vi "Parse StdErr for StdOut.vi"(11 "StdErr Event":string) -> (0 "error out":errorcluster, 2 "StdOut":string, 3 "StdErr":string)   [LabVIEW 2020, in "Kasli Wrapper 2.0.lvlib" / "Kasli Wrapper 2.0.lvclass"]
uses:
  Kasli Wrapper 2.0.lvclass
  <vilib>/regexp/Match Regular Expression.xnode
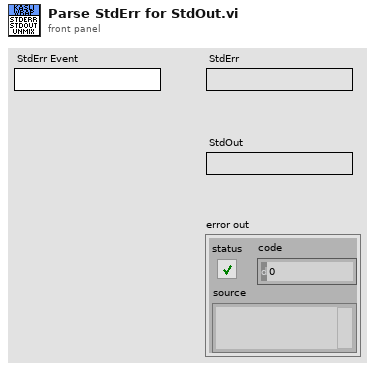
[diagram p1: front panel]
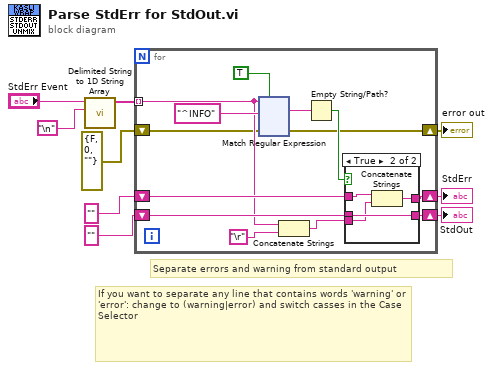
[diagram p0: block diagram]
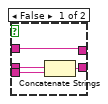
[diagram p2: hidden frame]
diagram:
  # "If you want to separate any line that contains words 'warning' or 'error': change to (warning|error) and switch casses in the Case Selector"
  # "Separate errors and warning from standard output"
  n1 = call <vilib>:"Delimited String to 1D String Array.vi"("delimiter"="\n", "delimited string"="StdErr Event") -> ("string array"=w7:string[])  [unwired: 9 in]
  n2 = for {
    tunnel: w7 -> [w14] mode=indexing
    shift-right: [w18] -> w3
    shift-left: "" -> [w19]
    shift-right: [w16] -> w4
    shift-left: "" -> [w15]
    shift-right: [w11] -> w9
    shift-left: errorcluster {"status"=FALSE, "code"=0, "source"=""} ("error out") -> [w10]
    n3 = xnode "Match Regular Expression"("input string"=w14, "regular expression"="^INFO", "error in"=w10, "ignore case? (F)"=TRUE) -> ("whole match"=w20:string, "error out"=w11:errorcluster)  [unwired: 2 in, 3 out]
    n4 = Concatenate Strings(w14, "\r") -> (w13:string)
    n5 = Empty String/Path?(string/path=w20) -> (empty?=w17:bool)
    n6 = case shown="True" w17 {
      tunnel: w19 -> [w26 w30]
      tunnel: w13 -> [w25 w29]
      tunnel: [w24 w30] -> w18
      tunnel: [w23 w28] -> w16
      tunnel: w15 -> [w23 w27]
      frame False {
        n7 = Concatenate Strings(w26, w25) -> (w24:string)
      }
      frame True {
        n8 = Concatenate Strings(w27, w29) -> (w28:string)
      }
    }
  }
  "error out" <- w9
  "StdErr" <- w4
  "StdOut" <- w3
